vi "Read_calibration_files.vi"() -> ()   [LabVIEW 2017]
uses:
  Controls/Pressure_Units.ctl
  Controls/Post_Process.ctl
  Controls/Instrument_Array.ctl
  Globals/Meas_global.vi
  Globals/Trav_pos_global.vi
  Acquisition/PWA/PWAtasksGLOBAL.vi
panel:
  in  "Pressure Units":T1
  # "This Program Read data in from the calibration files"
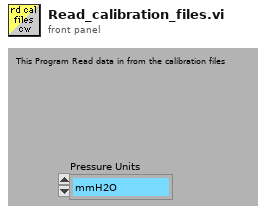
[diagram p1: front panel]
types:
  T1 = typedef "Pressure_Units.ctl" = enum16{"mmH2O", "mmHg", "Pa (N/m^2)", "mbar", "bar"}
  T2 = typedef "Analysis_info_cluster.ctl" = cluster{"Colour":u32, "Inst type":T3, "Inst name":string, "Symbol":string, "Code name":string, "Extra Info":string, "Inst Array":T4, "Extra Titles":string[], "Extra Values":string[], "U":dbl, "u^2":dbl, "u^3":dbl, "u^4":dbl, "Skew_u":dbl, "Kurt_u":dbl, "Sd Error in Mean":dbl, "% u'/U":dbl, "X":dbl, "Y":dbl, "Z":dbl, "Timescale integral Estimate":dbl, "Sd Error in Variance":dbl, "Calib File":path, "Calib Constants":dbl[], "Output Position":bool, "Full Stats":bool, "Av Sampling Rate":dbl, "Av No of Samples":dbl, "Total Meas Time (s)":dbl, "ADAM Ch Name":string, "Max value":dbl, "Min value":dbl, "Sync Delay Time (s)":dbl}
  T3 = typedef "Inst_type.ctl" = enum16{"Propeller anemometer", "Raw voltage", "Pressure Transducer", "Pitot-static tube", "Preston tube", "Hot wire", "Cross wire 1", "Cross wire 2", "Generic Linear", "Generic Polynomial", "Generic BackPoly", "Fast FID", "Thermocouple", "Cold wire", "Pulsed Wire", "LDA Vel", "LDA Tran time", "LDA Arr time", "Microphone"}
  T4 = typedef "Instrument_Array.ctl" = enum16{"PWA", "LDA", "Analogue"}
  T5 = typedef "PWA_Data.ctl" = enum16{"No PWA Data", "One Ch PWA"}
  T6 = typedef "Post_Process.ctl" = enum16{"Take New Data", "Post Process Raw Data File"}
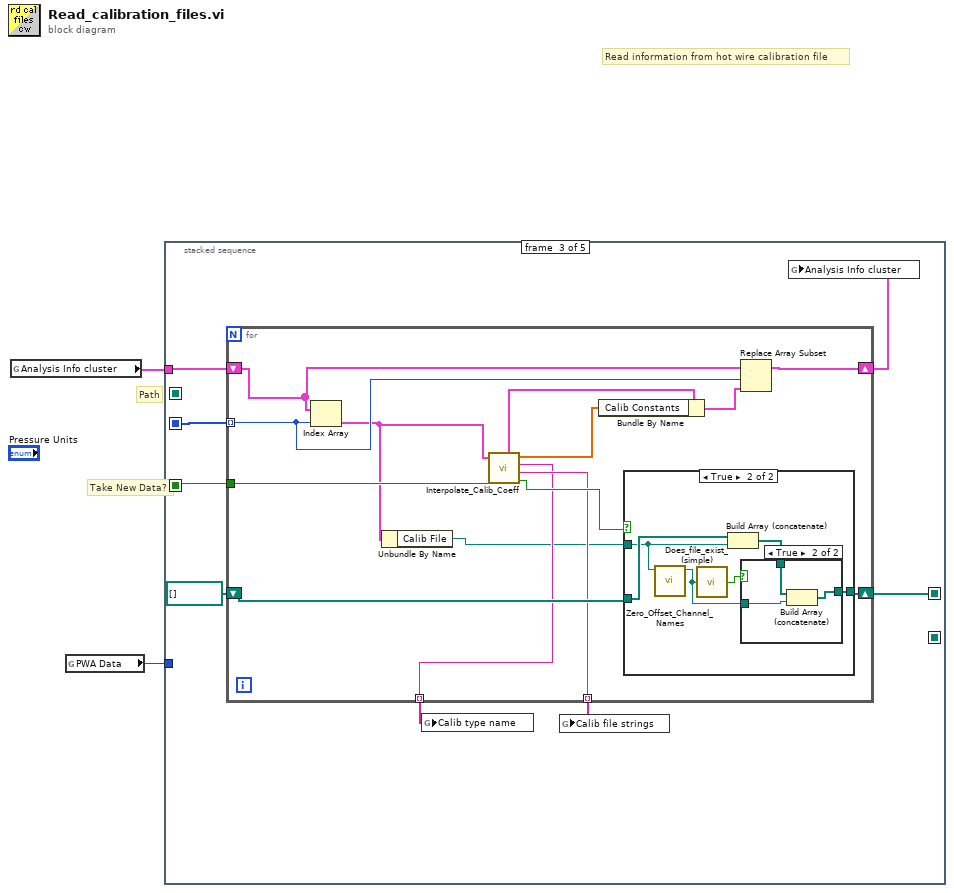
[diagram p0: block diagram]
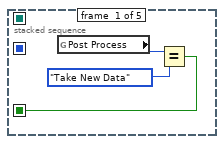
[diagram p2: hidden frame]
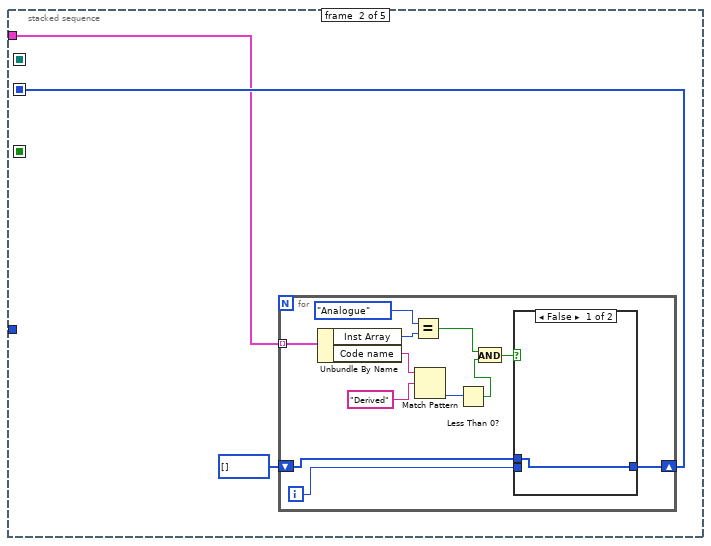
[diagram p3: hidden frame]
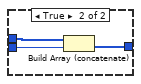
[diagram p4: hidden frame]
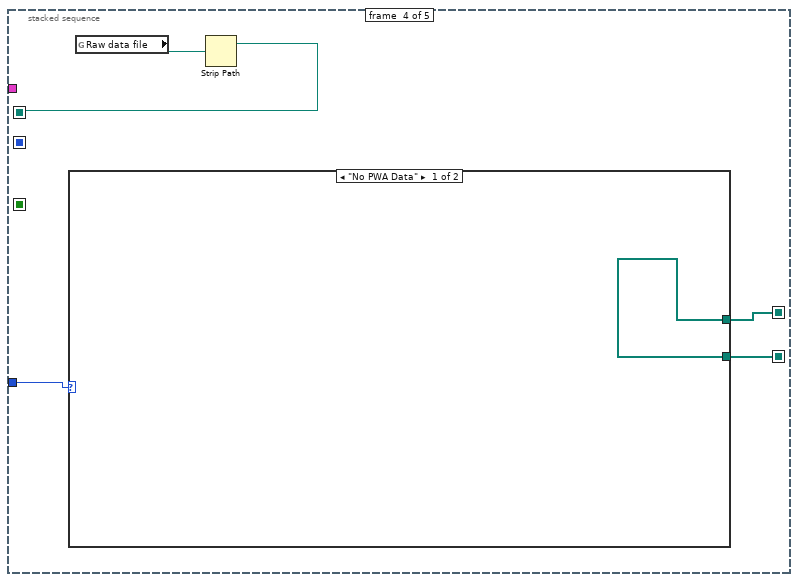
[diagram p7: hidden frame]
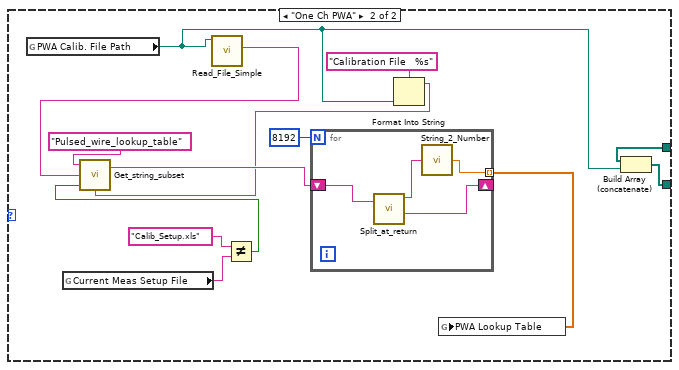
[diagram p8: hidden frame]
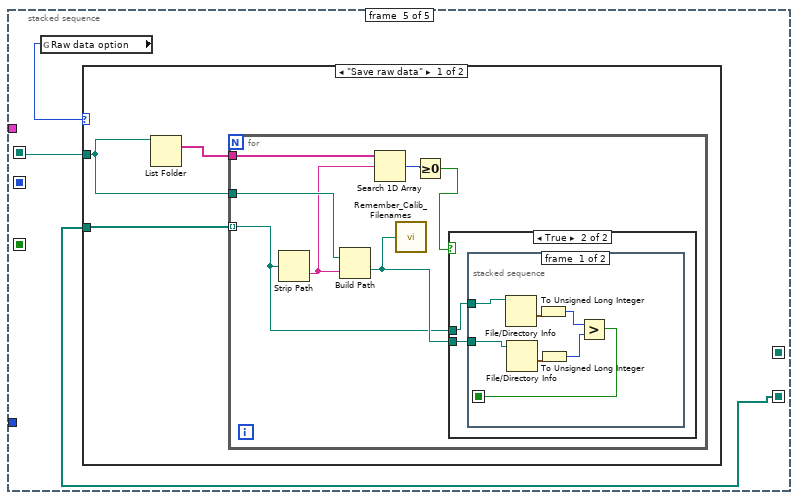
[diagram p9: hidden frame]
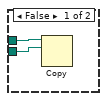
[diagram p10: hidden frame]
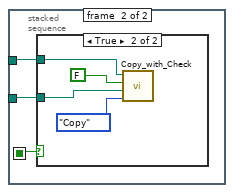
[diagram p11: hidden frame]
diagram:
  # "Take New Data?"
  # "Path"
  # "Read information from hot wire calibration file"
  n1 = global read "Meas_global.vi" "Analysis Info cluster"() -> (w1:T2[])
  n2 = global read "Meas_global.vi" "PWA Data"() -> (w2:T5)
  n3 = stacked-sequence {
    seq-local: [_ _ w32 _ _] -> [_ _ _ w58 _]
    seq-local: [_ _ _ w61 _] -> [_ _ _ _ w82]
    seq-local: [w3 _ _ _ _] -> [_ _ w30 _ _]
    seq-local: [_ _ _ w59 _] -> [_ _ _ _ w81]
    seq-local: [_ w7 _ _ _] -> [_ _ w26 _ _]
    tunnel: w2 -> [_ _ _ w60 _]
    tunnel: w1 -> [_ w6 w27 _ _]
    frame #0 {
      n4 = global read "Meas_global.vi" "Post Process"() -> (w4:T6)
      n5 = Equal?(x=w4, y=Post_Process."Take New Data" ("Post Process")) -> (x = y?=w3:bool)
    }
    frame #1 {
      n6 = for {
        tunnel: w6 -> [w12] mode=indexing
        shift-right: [w9] -> w7
        shift-left: i32[] [] -> [w10]
        i -> [w11]
        n7 = Unbundle By Name(w12) -> ("Inst Array"=w20:T4, "Code name"=w18:string)
        n8 = Equal?(x=Instrument_Array."Analogue" ("Inst Array"), y=w20) -> (x = y?=w14:bool)
        n9 = Match Pattern(string=w18, regular expression="Derived") -> (offset past match=w16:i32)  [unwired: 4 out]
        n10 = Less Than 0?(x=w16) -> (x < 0?=w15:bool)
        n11 = And(x=w14, y=w15) -> (x .and. y?=w13:bool)
        n12 = case shown="False" w13 {
          tunnel: w11 -> [_ w24]
          tunnel: w10 -> [w21 w23]
          tunnel: [w21 w22] -> w9
          frame False {
          }
          frame True {
            n13 = Build Array (concatenate)(w23, w24) -> (w22:i32[])
          }
        }
      }
    }
    frame #2 {
      n14 = for {
        shift-right: [w45] -> w32
        shift-left: path[] [] -> [w46]
        tunnel: w30 -> [w44]
        tunnel: [w42] -> w29 mode=indexing
        tunnel: [w41] -> w28 mode=indexing
        shift-right: [w38] -> w25
        shift-left: w27 -> [w40]
        tunnel: w26 -> [w39] mode=indexing
        n15 = Index Array(array=w40, index=w39) -> (element=w34:T2)
        n16 = Unbundle By Name(w34) -> ("Calib File"=w33:path)
        n17 = call "Interpolate_Calib_Coeff.vi"("Analysis Info cluster"=w34, "Take New Data?"=w44) -> ("Calib Coeff"=w35:dbl[], "Calib Type Name"=w41:string, "Calib file string"=w42:string, "Read file"=w43:bool, "Analysis Info cluster  Out"=w37:T2)  [unwired: 1 in]
        n18 = Bundle By Name(cluster=w37, "Calib Constants"=w35) -> (w36:T2)
        n19 = case shown="True" w43 {
          tunnel: w46 -> [w47 w53]
          tunnel: [w47 w48] -> w45
          tunnel: w33 -> [_ w52]
          frame False {
          }
          frame True {
            n20 = call "Zero_Offset_Channel_Names.vi"("Calib Filename"=w52) -> ("Zero Filename"=w49:path)  [unwired: 3 in, 3 out]
            n21 = call "Does_file_exist_(simple).vi"("Pathname"=w49) -> ("exists?"=w51:bool)
            n22 = Build Array (concatenate)(w53, w52) -> (w50:path[])
            n23 = case shown="True" w51 {
              tunnel: w50 -> [w54 w57]
              tunnel: w49 -> [_ w56]
              tunnel: [w54 w55] -> w48
              frame False {
              }
              frame True {
                n24 = Build Array (concatenate)(w57, w56) -> (w55:path[])
              }
            }
          }
        }
        n25 = Replace Array Subset(array=w40, new element=w36, index=w39) -> (w38:T2[])
      }
      n26 = global write "Meas_global.vi" "Calib type name"(w28) -> ()
      n27 = global write "Meas_global.vi" "Calib file strings"(w29) -> ()
      n28 = global write "Meas_global.vi" "Analysis Info cluster"(w25) -> ()
    }
    frame #3 {
      n29 = case shown="\"No PWA Data\"" w60 {
        tunnel: [w63 w67] -> w59
        tunnel: w58 -> [w63 w68]
        frame "No PWA Data" {
        }
        frame "One Ch PWA" {
          n30 = global read "PWAtasksGLOBAL.vi" "PWA Calib. File Path"() -> (w65:path)
          n31 = global read "Trav_pos_global.vi" "Current Meas Setup File"() -> (w75:string)
          n32 = call "Read_File_Simple.vi"("Filename"=w65) -> ("string"=w69:string)  [unwired: 2 in, 7 out]
          n33 = Not Equal?(x="Calib_Setup.xls", y=w75) -> (x != y?=w76:bool)
          n34 = Format Into String(format string="Calibration File   %s", w65) -> (resulting string=w64:string)  [unwired: 2 in, 1 out]
          n35 = call "Get_string_subset.vi"("String Name"=w64, "Show Dialog?"=w76, "String to split"=w69, "File Label"="Pulsed_wire_lookup_table") -> ("Output string"=w71:string)  [unwired: 1 out]
          n36 = for {
            N: 8192 -> [_]
            shift-right: [w79] -> _
            shift-left: w71 -> [w80]
            tunnel: [w77] -> w72 mode=indexing
            n37 = call "Split_at_return.vi"("String"=w80) -> ("before substring"=w78:string, "after substring"=w79:string)  [unwired: 1 in, 2 out]
            n38 = call "String_2_Number.vi"("Value"=w78) -> ("Numeric"=w77:dbl)
          }
          n39 = global write "PWAtasksGLOBAL.vi" "PWA Lookup Table"(w72) -> ()
          n40 = Build Array (concatenate)(w68, w65) -> (w67:path[])
        }
      }
      n41 = global read "Meas_global.vi" "Raw data file"() -> (w62:path)
      n42 = Strip Path(path=w62) -> (stripped path=w61:path)  [unwired: 1 out]
    }
    frame #4 {
      n43 = global read "Meas_global.vi" "Raw data option"() -> (w83:enum16{"Save raw data", "Raw data not saved"})
      n44 = case shown="\"Save raw data\"" w83 {
        tunnel: w81 -> [w86 _]
        tunnel: w82 -> [w84 _]
        frame "Save raw data" {
          n45 = List Folder(path=w84) -> (filenames=w85:string[])  [unwired: 1 in, 5 out]
          n46 = for {
            tunnel: w86 -> [w87] mode=indexing
            tunnel: w84 -> [w90]
            tunnel: w85 -> [w93]
            n47 = Strip Path(path=w87) -> (name=w89:string)  [unwired: 1 out]
            n48 = Build Path(base path=w90, name or relative path=w89) -> (appended path=w88:path)
            n49 = Search 1D Array(1D array=w93, element=w89) -> (index of element=w92:i32)  [unwired: 1 out]
            n50 = call "Remember_Calib_Filenames.vi"("Filename to Remember"=w88) -> ()  [unwired: 1 out]
            n51 = Greater Or Equal To 0?(x=w92) -> (x >= 0?=w91:bool)
            n52 = case shown="True" w91 {
              tunnel: w88 -> [w95 w96]
              tunnel: w87 -> [w94 w97]
              frame False {
                n53 = Copy(10:w95, 11:w94) -> ()  [unwired: 1 in, 5 out]
              }
              frame True {
                n54 = stacked-sequence {
                  seq-local: [w100 _] -> [_ w107]
                  tunnel: w97 -> [w104 w105]
                  tunnel: w96 -> [w103 w106]
                  frame #0 {
                    n55 = File/Directory Info(path=w104) -> (last mod=w98:timestamp)  [unwired: 1 in, 6 out]
                    n56 = File/Directory Info(path=w103) -> (last mod=w99:timestamp)  [unwired: 1 in, 6 out]
                    n57 = To Unsigned Long Integer(number=w98) -> (unsigned 32bit integer=w102:u32)
                    n58 = To Unsigned Long Integer(number=w99) -> (unsigned 32bit integer=w101:u32)
                    n59 = Greater?(x=w102, y=w101) -> (0:w100:bool)
                  }
                  frame #1 {
                    n60 = case shown="True" w107 {
                      tunnel: w106 -> [_ w110]
                      tunnel: w105 -> [_ w111]
                      frame False {
                      }
                      frame True {
                        n61 = call "Copy_with_Check.vi"("Mode"=enum16{"Move", "Copy"}."Copy", "Target Path"=w110, "Variable Target?"=FALSE, "Source Path"=w111) -> ()  [unwired: 1 out]
                      }
                    }
                  }
                }
              }
            }
          }
        }
        frame "Raw data not saved" {
        }
      }
    }
  }
